vi "Sort Class Array for Tree.vi"(11 "All Classes":T2(array[cluster])) -> (3 "All Classes Tree Sorted":T1(array[cluster]))   [LabVIEW 2023]
uses:
  <userlib>/_OpenG.lib/comparison/comparison.llb/String Changed__ogtk.vi
panel:
  out "size(s)":i32
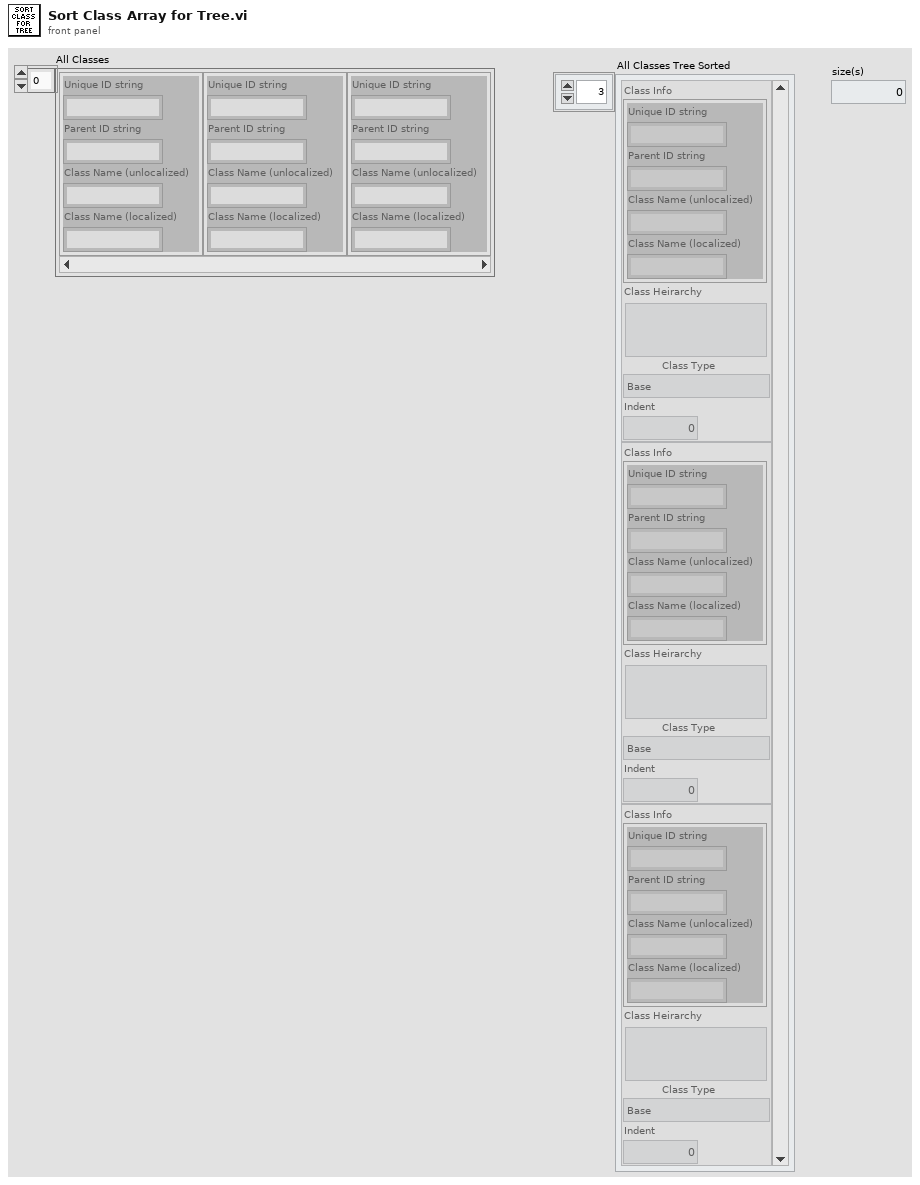
[diagram p1: front panel]
types:
  T1 = cluster{"Class Info":cluster{"Unique ID string":string, "Parent ID string":string, "Class Name (unlocalized)":string, "Class Name (localized)":string}, "Class Heirarchy":string, "Class Type":enum16{"Unknown", "Base", "Scripting", "Private", "Deprecated", "None", "Divider"}, "Indent":u32}[]
  T2 = cluster{"Unique ID string":string, "Parent ID string":string, "Class Name (unlocalized)":string, "Class Name (localized)":string}[]
  T3 = cluster{"Unique ID string":string, "Parent ID string":string, "Class Name (unlocalized)":string, "Class Name (localized)":string}
  T4 = cluster{cluster{"Unique ID string":string, "Parent ID string":string, "Class Name (unlocalized)":string, "Class Name (localized)":string}[]}
  T5 = cluster{"Class Name (unlocalized)":string, "Property/Method Info":cluster{"Unique ID string":string, "Parent ID string":string, "Class Name (unlocalized)":string, "Class Name (localized)":string}}
  T6 = cluster{"Class Name (unlocalized)":string, "Property/Method Info":cluster{"Unique ID string":string, "Parent ID string":string, "Class Name (unlocalized)":string, "Class Name (localized)":string}}[]
  T7 = cluster{cluster{"Unique ID string":string, "Parent ID string":string, "Class Name (unlocalized)":string, "Class Name (localized)":string}[]}[]
  T8 = cluster{"Class Info":cluster{"Unique ID string":string, "Parent ID string":string, "Class Name (unlocalized)":string, "Class Name (localized)":string}, "Class Heirarchy":string, "Class Type":enum16{"Unknown", "Base", "Scripting", "Private", "Deprecated", "None", "Divider"}, "Indent":u32}
  T9 = enum16{"Unknown", "Base", "Scripting", "Private", "Deprecated", "None", "Divider"}
  T10 = cluster{"Class Info":cluster{"Unique ID string":string, "Parent ID string":string, "Class Name (unlocalized)":string, "Class Name (localized)":string}, "Class Heirarchy":string, "Property Type":enum16{"Unknown", "Base", "Scripting", "Private", "Deprecated", "None", "Divider"}, "Indent":u32}[]
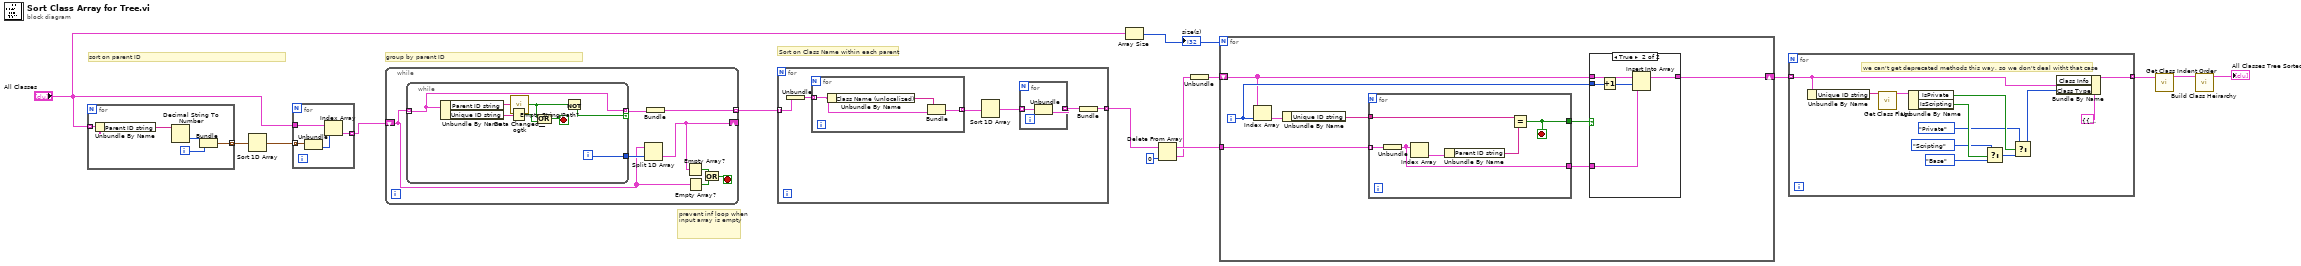
[diagram p0: block diagram]
diagram:
  # "prevent inf loop when input array is empty"
  # "Sort on Class Name within each parent"
  # "group by parent ID"
  # "sort on parent ID"
  n1 = for {
    tunnel: "All Classes" -> [w19] mode=indexing
    tunnel: [w16] -> w6 mode=indexing
    i -> [w17]
    n2 = Unbundle By Name(w19) -> ("Parent ID string"=w20:string)
    n3 = Decimal String To Number(string=w20) -> (number=w18:i32)  [unwired: 2 in, 1 out]
    n4 = Bundle(w18, w17) -> (w16:cluster{i32, i32})  [unwired: 1 in]
  }
  n5 = Sort 1D Array(array=w6) -> (sorted array=w5:cluster{i32, i32}[])
  n6 = for {
    tunnel: w5 -> [w23] mode=indexing
    tunnel: "All Classes" -> [w24]
    tunnel: [w21] -> w3 mode=indexing
    n7 = Unbundle(w23) -> (w22:i32)  [unwired: 1 out]
    n8 = Index Array(array=w24, index=w22) -> (element=w21:T3)
  }
  n9 = while {
    shift-right: [w29] -> _
    shift-left: w3 -> [w28]
    tunnel: [w31] -> w15 mode=indexing
    stop <- w25 stop-if-true
    n10 = while {
      tunnel: [w37] -> w32 mode=indexing if=w40
      tunnel: w28 -> [w37] mode=indexing
      tunnel: [w39] -> w30
      i -> [w39]
      stop <- w34 stop-if-true
      n11 = Unbundle By Name(w37) -> ("Parent ID string"=w38:string, "Unique ID string"=w36:string)
      n12 = Empty String/Path?(string/path=w36) -> (empty?=w35:bool)
      n13 = call-poly <userlib>:"Data Changed__ogtk.vi"("String"=w38) -> ("Changed"=w33:bool)
      n14 = Compound Arithmetic op=OR(w33, w35) -> (w34:bool)
      n15 = Not(x=w33) -> (.not. x?=w40:bool)
    }
    n16 = Split 1D Array(array=w28, index=w30) -> (second subarray=w29:T2)  [unwired: 1 out]
    n17 = Bundle(w32) -> (w31:T4)  [unwired: 1 in]
    n18 = Empty Array?(array=w29) -> (empty?=w26:bool)
    n19 = Empty Array?(array=w28) -> (empty?=w27:bool)
    n20 = Compound Arithmetic op=OR(w26, w27) -> (w25:bool)
  }
  n21 = for {
    tunnel: w15 -> [w46] mode=indexing
    tunnel: [w41] -> w14 mode=indexing
    n22 = Unbundle(w46) -> (w45:T2)
    n23 = for {
      tunnel: [w51] -> w44 mode=indexing
      tunnel: w45 -> [w50] mode=indexing
      n24 = Unbundle By Name(w50) -> ("Class Name (unlocalized)"=w49:string)
      n25 = Bundle("Class Name (unlocalized)"=w49, "Property/Method Info"=w50) -> (w51:T5)  [unwired: 1 in]
    }
    n26 = Sort 1D Array(array=w44) -> (sorted array=w43:T6)
    n27 = for {
      tunnel: w43 -> [w48] mode=indexing
      tunnel: [w47] -> w42 mode=indexing
      n28 = Unbundle(w48) -> ("Property/Method Info"=w47:T3)  [unwired: 1 out]
    }
    n29 = Bundle(w42) -> (w41:T4)  [unwired: 1 in]
  }
  n30 = Array Size(array="All Classes") -> (size(s)=w9:i32)
  "size(s)" <- w9
  n31 = Delete From Array(array=w14, index=0) -> (deleted portion=w11:T4, array with subset deleted=w12:T7)  [unwired: 1 in]
  n32 = Unbundle(w11) -> (w10:T2)
  n33 = for {
    N: w9 -> [_]
    shift-right: [w53] -> w8
    shift-left: w10 -> [w54]
    tunnel: w12 -> [w58]
    i -> [w55]
    n34 = Index Array(array=w54, index=w55) -> (element=w59:T3)
    n35 = Unbundle By Name(w59) -> ("Unique ID string"=w57:string)
    n36 = for {
      tunnel: w58 -> [w71] mode=indexing
      tunnel: w57 -> [w69]
      tunnel: [w67] -> w56
      tunnel: [w66] -> w52
      stop <- w66 stop-if-true
      n37 = Unbundle(w71) -> (w67:T2)
      n38 = Index Array(array=w67) -> (element=w70:T3)  [unwired: 1 in]
      n39 = Unbundle By Name(w70) -> ("Parent ID string"=w68:string)
      n40 = Equal?(x=w69, y=w68) -> (x = y?=w66:bool)
    }
    n41 = case shown="True" w52 {
      tunnel: w56 -> [_ w65]
      tunnel: w55 -> [_ w64]
      tunnel: w54 -> [w60 w63]
      tunnel: [w60 w62] -> w53
      frame False {
      }
      frame True {
        n42 = Increment(x=w64) -> (x+1=w61:i32)
        n43 = Insert Into Array(array=w63, index=w61, new element=w65) -> (w62:T2)
      }
    }
  }
  n44 = for {
    tunnel: w8 -> [w72] mode=indexing
    tunnel: [w74] -> w7 mode=indexing
    # "we can't get deprecated methods this way, so we don't deal witht that case"
    n45 = Unbundle By Name(w72) -> ("Unique ID string"=w83:string)
    n46 = call "Get Class Flags.vi"("Class ID"=w83) -> ("Flags"=w82:cluster{"IsPrivate":bool, "IsScripting":bool})  [unwired: 9 in, 1 out]
    n47 = Unbundle By Name(w82) -> ("IsPrivate"=w77:bool, "IsScripting"=w80:bool)
    n48 = Select(t=T9."Scripting" ("Property Type"), s=w80, f=T9."Base" ("Property Type")) -> (s? t:f=w78:T9)
    n49 = Select(t=T9."Private" ("Property Type"), s=w77, f=w78) -> (s? t:f=w75:T9)
    n50 = Bundle By Name(cluster=T8 {"Class Info"={"Unique ID string"="", "Parent ID string"="", "Class Name (unlocalized)"="", "Class Name (localized)"=""}, "Class Heirarchy"="", "Class Type"=enum."Base", "Indent"=0} ("Property/Method Info"), "Class Info"=w72, "Class Type"=w75) -> (w74:T8)
  }
  n51 = call "Get Class Indent Order.vi"("Tree Sorted Array"=w7) -> ("Tree Sorted Array Out"=w2:T1)  [unwired: 9 in, 1 out]
  n52 = call "Build Class Heirarchy.vi"("Classes In"=w2) -> ("Classes Out"=→"All Classes Tree Sorted":T10)  [unwired: 10 in]
